vi "Get VI Indicators.vi"(10 "DataType":string(combo)="error", 11 "VI ref.":refnum<vi>) -> (2 "#indicators":i32, 3 "Controls Array":refnum<vi>[](array[refnum]))   [LabVIEW 2014]
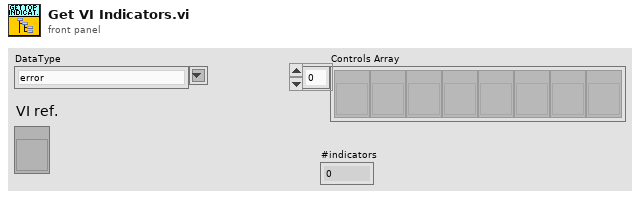
[diagram p1: front panel]
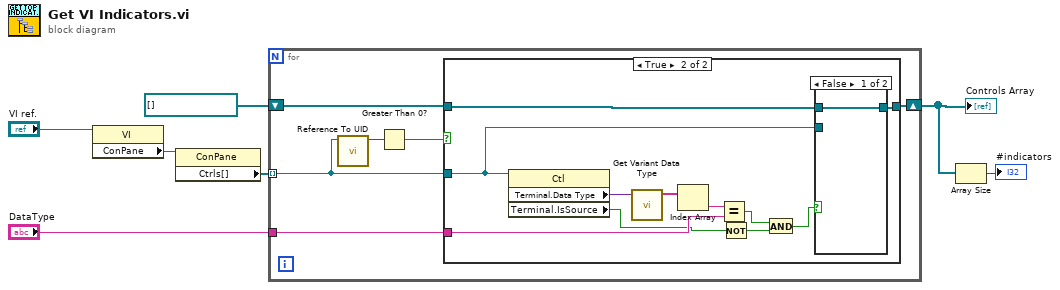
[diagram p0: block diagram]
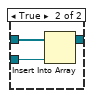
[diagram p3: hidden frame]
diagram:
  n1 = property class="VI"(reference="VI ref.") -> ("ConPane"=w7:refnum<vi>)  [unwired: 1 in, 2 out]
  n2 = property class="ConPane"(reference=w7) -> ("Ctrls[]"=w6:refnum<vi>[])  [unwired: 1 in, 2 out]
  n3 = for {
    tunnel: w6 -> [w10] mode=indexing
    tunnel: "DataType" -> [w13]
    shift-right: [w11] -> w4
    shift-left: refnum<vi>[] [] -> [w12]
    n4 = call "Reference To UID.vi"("Reference"=w10) -> ("UID"=w9:i32)  [unwired: 10 in]
    n5 = Greater Than 0?(x=w9) -> (x > 0?=w8:bool)
    n6 = case shown="True" w8 {
      tunnel: w13 -> [_ w22]
      tunnel: w12 -> [w14 w21]
      tunnel: w10 -> [_ w20]
      tunnel: [w14 w19] -> w11
      frame False {
      }
      frame True {
        n7 = property class="Ctl"(reference=w20) -> ("Terminal.Data Type"=w25:variant, "Terminal.IsSource"=w16:bool)  [unwired: 1 in, 2 out]
        n8 = call "Get Variant Data Type.vi"("variant"=w25) -> ("Data Type"=w24:string[])  [unwired: 10 in]
        n9 = Index Array(array=w24) -> (element=w23:string)  [unwired: 1 in]
        n10 = Equal?(x=w23, y=w22) -> (x = y?=w18:bool)
        n11 = Not(x=w16) -> (.not. x?=w15:bool)
        n12 = And(x=w18, y=w15) -> (x .and. y?=w17:bool)
        n13 = case shown="False" w17 {
          tunnel: w21 -> [w26 w29]
          tunnel: w20 -> [_ w28]
          tunnel: [w26 w27] -> w19
          frame False {
          }
          frame True {
            n14 = Insert Into Array(array=w29, new element=w28) -> (w27:refnum<vi>[])  [unwired: 1 in]
          }
        }
      }
    }
  }
  "Controls Array" <- w4
  n15 = Array Size(array=w4) -> (size(s)=→"#indicators":i32)
